vi "ProdaNG.Oracle.FindPath.vi"(8 "error in (no error)":errorcluster) -> (0 "error out":errorcluster, 1 "found":bool, 2 "Tnsnames path":path)   [LabVIEW 2016]
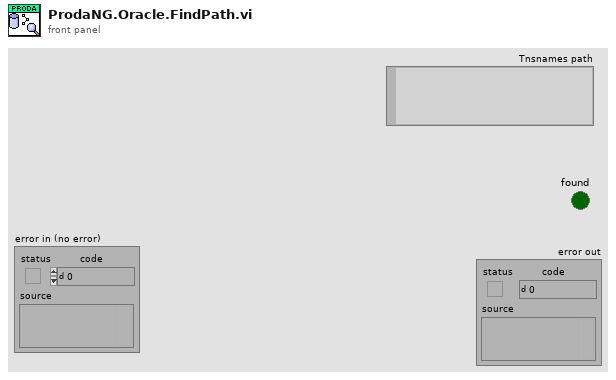
[diagram p1: front panel]
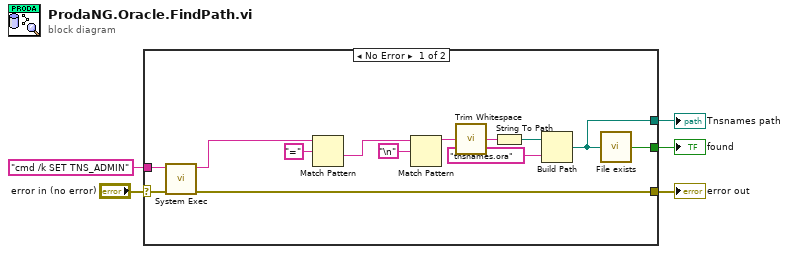
[diagram p0: block diagram]
diagram:
  n1 = case shown="No Error" "error in (no error)" {
    selector: "error in (no error)" -> [w17 w19]
    tunnel: "cmd /k SET TNS_ADMIN" ("command line") -> [w18 _]
    tunnel: [w16 w19] -> w4
    tunnel: [w10 _] -> w2
    tunnel: [w9 _] -> w1
    frame No Error {
      n2 = call <vilib>:"System Exec.vi"("error in (no error)"=w17, "command line"=w18) -> ("error out"=w16:errorcluster, "standard output"=w8:string)  [unwired: 6 in, 2 out]
      n3 = Match Pattern(string=w8, regular expression="=") -> (after substring=w6:string)  [unwired: 1 in, 3 out]
      n4 = Match Pattern(string=w6, regular expression="\n") -> (before substring=w14:string)  [unwired: 1 in, 3 out]
      n5 = call <vilib>:"Trim Whitespace.vi"("string"=w14) -> ("trimmed string"=w13:string)  [unwired: 1 in]
      n6 = String To Path(string=w13) -> (path=w12:path)
      n7 = Build Path(base path=w12, name or relative path="tnsnames.ora") -> (appended path=w10:path)
      n8 = call "File exists.vi"("file path"=w10) -> ("exists?"=w9:bool)  [unwired: 4 in]
    }
    frame Error {
    }
  }
  "error out" <- w4
  "found" <- w1
  "Tnsnames path" <- w2
